vi "ReadIPR.vi"(8 "error in":errorcluster, 9 "id_in":i32, 11 "connection ID":refnum<k5>) -> (0 "error out":errorcluster, 1 "Data out":string, 2 "IPR value":i32, 3 "connection ID out":refnum<k5>, 5 "id_out":i32)   [LabVIEW 2012]
doc: "This VI sends a trigger signal to the AWG and returns the IPR number. It is necessary to specify a delay value (longer than # of burst pulses x frequency) to read the correct IPR value."
panel:
  out "Data out 2":string
  out "Numeric":i32
  out "bytes written":i32
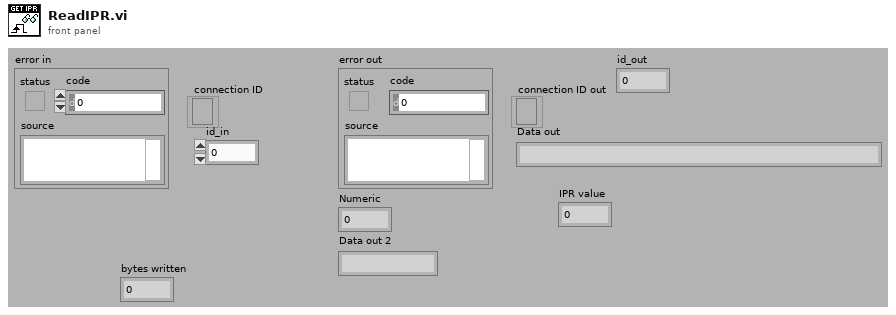
[diagram p1: front panel]
types:
  T1 = enum16{"Standard", "Buffered", "CRLF", "Immediate"}
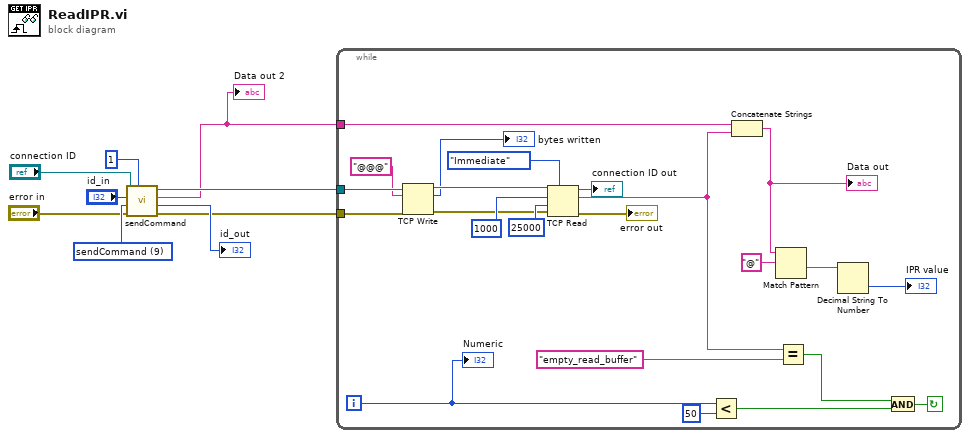
[diagram p0: block diagram]
diagram:
  w8 = u16 9 items=["sendCommand"=9, "FPGA_writeRegister"=3, "FPGA_readRegister"=2, "uC_writeRegister"=1, "uC_readRegister"=0] ("Action")
  n1 = call "sendCommand.vi"("Data"=1, "error in"="error in", "Action"=w8, "id_in"="id_in", "connection ID"="connection ID") -> ("error out"=w4:errorcluster, "id_out"=→"id_out":i32, "Data out"=w1:string, "connection ID out"=w3:refnum<k5>)  [unwired: 2 in, 1 out]
  "Data out 2" <- w1
  n2 = while {
    tunnel: w4 -> [w23]
    tunnel: w3 -> [w22]
    tunnel: w1 -> [w11]
    i -> [w15]
    stop <- w16 continue-if-true
    n3 = TCP Write(connection ID=w22, data in="@@@", error in (no error)=w23) -> (connection ID out=w27:refnum<k5>, bytes written=→"bytes written":i32, error out=w24:errorcluster)  [unwired: 1 in]
    n4 = TCP Read(connection ID=w27, bytes to read=1000, error in (no error)=w24, 7:T1."Immediate" ("mode (standard)"), 9:25000 ("timeout ms (25000)")) -> (connection ID out=→"connection ID out":refnum<k5>, data out=w12:string, error out=→"error out":errorcluster)
    n5 = Less?(x=w15, y=50) -> (x < y?=w13:bool)
    n6 = Concatenate Strings(w11, w12) -> (w10:string)
    "Data out" <- w10
    n7 = Match Pattern(string=w10, regular expression="@" ("search string/char (-)")) -> (after substring=w32:string)  [unwired: 1 in, 3 out]
    n8 = Equal?(x=w12, y="empty_read_buffer") -> (x = y?=w17:bool)
    n9 = Decimal String To Number(string=w32) -> (number=→"IPR value":i32)  [unwired: 2 in, 1 out]
    n10 = And(x=w17, y=w13) -> (x .and. y?=w16:bool)
    "Numeric" <- w15
  }
